vi "test.vi"() -> ()   [LabVIEW 2023]
uses:
  OWON SDS1022/OWON SDS1022.lvclass
  OWON SDS1022/Configurations/Voltmeter CFG/Voltmeter CFG.lvclass
panel:
  out "Avg Voltage Chart":dbl(graph)
  out "Iter Time":dbl
  in  "stop":bool
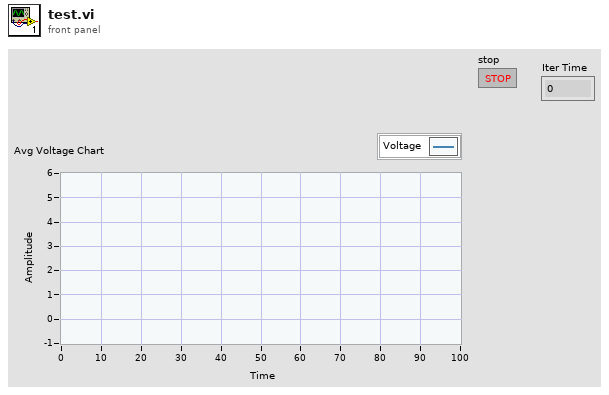
[diagram p1: front panel]
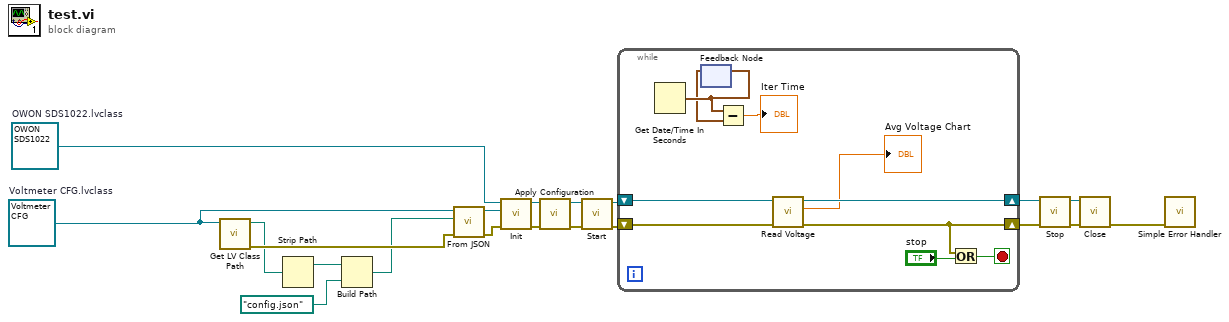
[diagram p0: block diagram]
diagram:
  w19 = refnum<class "Voltmeter CFG.lvclass"> refnum  # Voltmeter CFG.lvclass
  w18 = refnum<class "OWON SDS1022.lvclass"> refnum  # OWON SDS1022.lvclass
  n1 = call <vilib>:"Get LV Class Path.vi"("object"=w19) -> ("error out"=w16:errorcluster, "class path"=w14:path)  [unwired: 9 in]
  n2 = Strip Path(path=w14) -> (stripped path=w13:path)  [unwired: 1 out]
  n3 = Build Path(base path=w13, name or relative path=path "config.json") -> (appended path=w15:path)
  n4 = call-dynamic "From JSON.vi"("error in (no error)"=w16, "JSON Config"=w15, "object in"=w19) -> ("error out"=w11:errorcluster, "object out"=w12:refnum<class "Voltmeter CFG.lvclass">)  [unwired: 7 in]
  n5 = call-dynamic "Init.vi"("Error In"=w11, "IConfigure"=w12, "object in"=w18) -> ("Error Out"=w10:errorcluster, "object out"=w9:refnum<class "OWON SDS1022.lvclass">)  [unwired: 7 in]
  n6 = call-dynamic "Apply Configuration.vi"("error in"=w10, "Scope Base in"=w9) -> ("error out"=w8:errorcluster, "Scope Base out"=w2:refnum<class "OWON SDS1022.lvclass">)  [unwired: 8 in]
  n7 = call-dynamic "Start.vi"("Error In"=w8, "object in"=w2) -> ("Error Out"=w3:errorcluster, "object out"=w1:refnum<class "OWON SDS1022.lvclass">)  [unwired: 8 in]
  n8 = while {
    shift-right: [w22] -> w7
    shift-left: w3 -> [w30]
    shift-right: [w23] -> w6
    shift-left: w1 -> [w29]
    stop <- w24 stop-if-true
    n9 = Get Date/Time In Seconds() -> (seconds since 1Jan1904=w27:timestamp)
    n10 = feedback-in #1(w27) -> ()
    n11 = feedback #1() -> (w26:timestamp)  [unwired: 1 in]
    n12 = Subtract(x=w27, y=w26) -> (x-y=→"Iter Time":dbl)
    n13 = call-dynamic "Read Voltage.vi"("error in"=w30, "Scope Base in"=w29) -> ("error out"=w22:errorcluster, "Voltage"=→"Avg Voltage Chart":dbl, "Scope Base out"=w23:refnum<class "OWON SDS1022.lvclass">)  [unwired: 7 in]
    n14 = Or(x=w22, y="stop") -> (x .or. y?=w24:bool)
  }
  n15 = call-dynamic "Stop.vi"("Error In"=w7, "object in"=w6) -> ("Error Out"=w5:errorcluster, "object out"=w4:refnum<class "OWON SDS1022.lvclass">)  [unwired: 8 in]
  n16 = call-dynamic "Close.vi"("Error In"=w5, "object in"=w4) -> ("Error Out"=w20:errorcluster)  [unwired: 8 in, 1 out]
  n17 = call <vilib>:"Simple Error Handler.vi"("error in (no error)"=w20) -> ()  [unwired: 4 in, 5 out]
